vi "Start.vi"(0 "reference in":refnum<class "Speed.lvclass">, 5 "error in (no error)":errorcluster) -> (14 "reference out":refnum<class "Speed.lvclass">, 19 "error out":errorcluster)   [LabVIEW 2013, in "Speed.lvclass"]
uses:
  Speed.lvclass
  Dec_class/Dec.lvclass
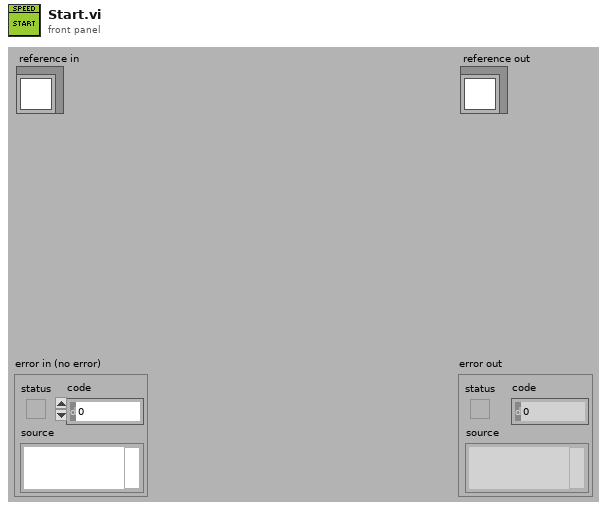
[diagram p1: front panel]
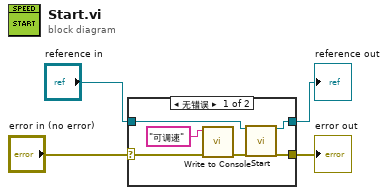
[diagram p0: block diagram]
diagram:
  n1 = case shown="无错误" "error in (no error)" {
    selector: "error in (no error)" -> [w8 w12]
    tunnel: [w5 w12] -> w3
    tunnel: [w7 w11] -> w1
    tunnel: "reference in" -> [w10 w11]
    frame No Error {
      n2 = call "Write to Console.vi"("error in (no error)"=w8, "Input"="可调速") -> ("error out"=w6:errorcluster)  [unwired: 9 in]
      n3 = call-parent "Start.vi"("reference in"=w10, "error in (no error)"=w6) -> ("reference out"=w7:refnum<class "Speed.lvclass">, "error out"=w5:errorcluster)  [unwired: 16 in]
    }
    frame Error {
    }
  }
  "error out" <- w3
  "reference out" <- w1
